vi "Substitute Constants.vi"(8 "Formula In":string, 10 "Data In":T1) -> (0 "Formula Out":string, 1 "Variables Out":string[](array[string]), 2 "Values Out":dbl[](array[numeric]))   [LabVIEW 2012, in "Calculator XControl.xctl"]
doc: "Substitute variable names such as pi, ans, and e with corresponding values."
uses:
  Calculator XControl.xctl
  Data 1.ctl
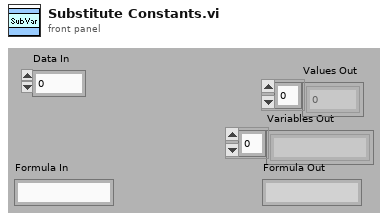
[diagram p1: front panel]
types:
  T1 = typedef "Calculator XControl.xctl/Data 1.ctl" = dbl
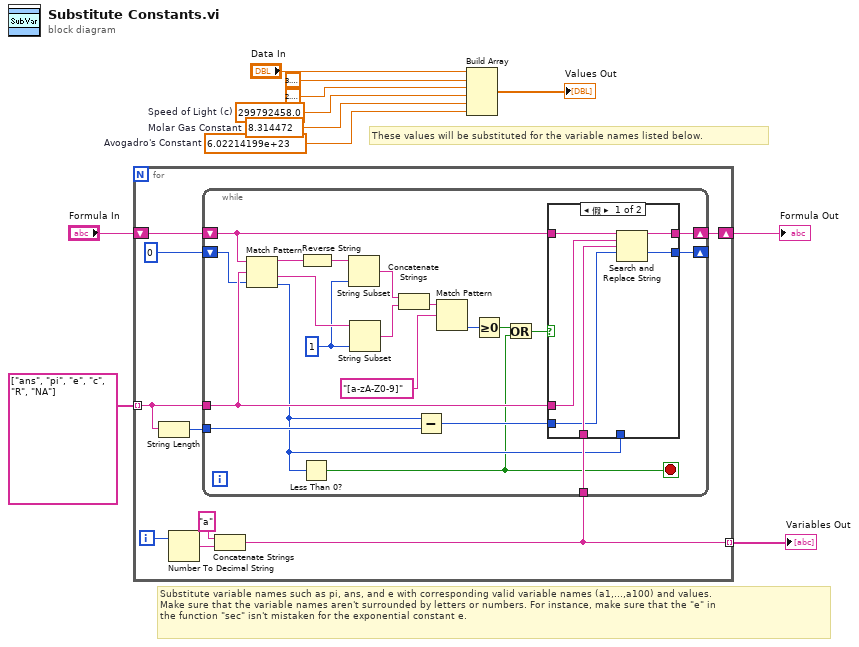
[diagram p0: block diagram]
diagram:
  w1 = 6.02214199e+23  # Avogadro's Constant
  w2 = 8.314472  # Molar Gas Constant
  w3 = 299792458.0  # Speed of Light (c)
  # "These values will be substituted for the variable names listed below."
  # "Substitute variable names such as pi, ans, and e with corresponding valid variable names (a1,...,a100) and values.\nMake sure that the variable names aren't surrounded by letters or numbers. For instance, make sure that the \"e\" in\nthe function \"sec\" isn't mistaken for the exponential constant e."
  n1 = for {
    tunnel: string[] ["ans", "pi", "e", "c", "R", "NA"] ("Variables Out") -> [w13] mode=indexing
    shift-right: [w16] -> w5
    shift-left: "Formula In" -> [w17]
    tunnel: [w15] -> w4 mode=indexing
    i -> [w20]
    n2 = String Length(string=w13) -> (length=w12:i32)
    n3 = Number To Decimal String(number=w20) -> (decimal integer string=w19:string)  [unwired: 1 in]
    n4 = Concatenate Strings("a" ("string"), w19) -> (w15:string)
    n5 = while {
      shift-right: [w33] -> w16
      shift-left: w17 -> [w34]
      tunnel: w15 -> [w31]
      tunnel: w13 -> [w32]
      shift-right: [w30] -> _
      shift-left: 0 ("offset past replacement") -> [w29]
      tunnel: w12 -> [w28]
      stop <- w22 stop-if-true
      w25 = 1 ("length (rest)")
      n6 = Match Pattern(string=w34, regular expression=w32, offset (0)=w29) -> (before substring=w41:string, after substring=w40:string, offset past match=w24:i32)  [unwired: 1 out]
      n7 = Less Than 0?(x=w24) -> (x < 0?=w22:bool)
      n8 = Reverse String(1:w41) -> (0:w26:string)
      n9 = String Subset(string=w26, length (rest)=w25) -> (substring=w39:string)  [unwired: 1 in]
      n10 = String Subset(string=w40, length (rest)=w25) -> (substring=w38:string)  [unwired: 1 in]
      n11 = Concatenate Strings(w39, w38) -> (w37:string)
      n12 = Subtract(x=w24, y=w28) -> (x-y=w27:i32)
      n13 = Match Pattern(string=w37, regular expression="[a-zA-Z0-9]") -> (offset past match=w35:i32)  [unwired: 1 in, 3 out]
      n14 = Greater Or Equal To 0?(x=w35) -> (x >= 0?=w23:bool)
      n15 = Or(x=w23, y=w22) -> (x .or. y?=w21:bool)
      n16 = case shown="假" w21 {
        tunnel: w34 -> [w47 w49]
        tunnel: [w46 w49] -> w33
        tunnel: w32 -> [w44 _]
        tunnel: w31 -> [w45 _]
        tunnel: [w43 w48] -> w30
        tunnel: w27 -> [w42 _]
        tunnel: w24 -> [_ w48]
        frame False {
          n17 = Search and Replace String(input string=w47, search string=w44, replace string=w45, offset=w42) -> (result string=w46:string, offset past replacement=w43:i32)  [unwired: 4 in, 2 out]
        }
        frame True {
        }
      }
    }
  }
  "Variables Out" <- w4
  "Formula Out" <- w5
  n18 = Build Array("Data In", 3.141592653589793, 2.718281828459045, w3, w2, w1) -> (→"Values Out":T1[])
